vi "Deadzone.vi"(1 "Input":dbl) -> (0 "Output":dbl)   [LabVIEW 2015]
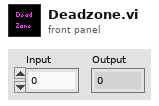
[diagram p1: front panel]
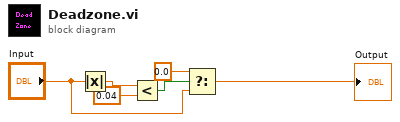
[diagram p0: block diagram]
diagram:
  n1 = Absolute Value(x="Input") -> (abs(x)=w6:dbl)
  n2 = Less?(x=w6, y=0.04) -> (x < y?=w4:bool)
  n3 = Select(t=0.0, s=w4, f="Input") -> (s? t:f=→"Output":dbl)
